vi "Real LU Factorization.vi"(0 "A":T1) -> (1 "L":T1, 2 "U":T1, 3 "P":i32[][](array[numeric]), 4 "error":i32)   [LabVIEW 2014, in "NI_AALPro.lvlib"]
doc: "Performs the LU factorization of <B>A</B> so that <B>PA</B> = <B>LU</B>. Wire data to the <B>A</B> input to determine the polymorphic instance to use or manually select the instance."
uses:
  NI_AALPro.lvlib
  RealMatrix.ctl
  NI_AALBase.lvlib
  NI_Matrix.lvlib
panel:
  # "LU Factorization"
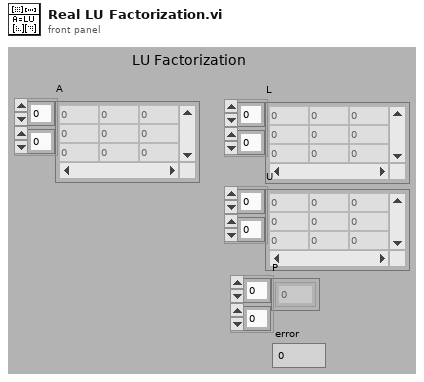
[diagram p1: front panel]
types:
  T1 = typedef "NI_Matrix.lvlib/RealMatrix.ctl" = dbl[][]
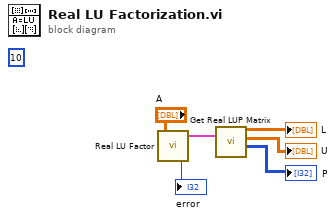
[diagram p0: block diagram]
diagram:
  (unwired) 10
  n1 = call "Real LU Factor.vi"("A"="A") -> ("LU Info"=w5:cluster{"LU":dbl[][], "Pivot":i32[]}, "error"=→"error":i32)  [unwired: 1 out]
  n2 = call "Get Real LUP Matrix.vi"("LU Info"=w5) -> ("L"=→"L":T1, "U"=→"U":T1, "P"=→"P":i32[][])  [unwired: 1 in]
